vi "oa_Reset if Parameters Change for Triggered Even Angle Signal (N Channels).vi"(7 "reset? (T)":bool=TRUE, 8 "block size":i32=-1, 9 "trigger period [rev]":dbl=1.0, 11 "even angle signals":cluster{"r0":dbl, "dr":dbl, "Y":dbl[]}[](array[cluster]) {"r0" format="%.2p"; "dr" format="%.2p"; "Y" format="%.2f"}) -> (0 "block size out":i32, 1 "trigger period out [rev]":dbl, 3 "even angle signals out":cluster{"r0":dbl, "dr":dbl, "Y":dbl[]}[](array[cluster]) {"r0" format="%.2p"; "dr" format="%.2p"; "Y" format="%.2f"}, 5 "reset out":bool)   [LabVIEW 2017, in "SoundVib_OAUtility.lvlib"]
uses:
  <vilib>/addons/Sound and Vibration/Order Analysis/Utility/SoundVib_OAUtility.lvlib
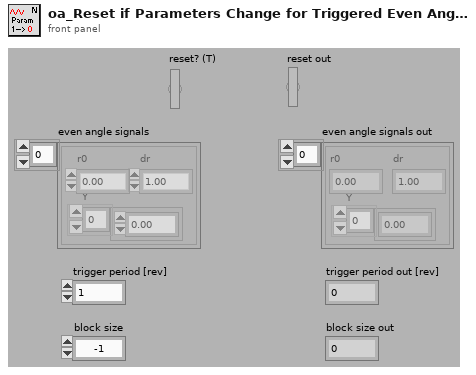
[diagram p1: front panel]
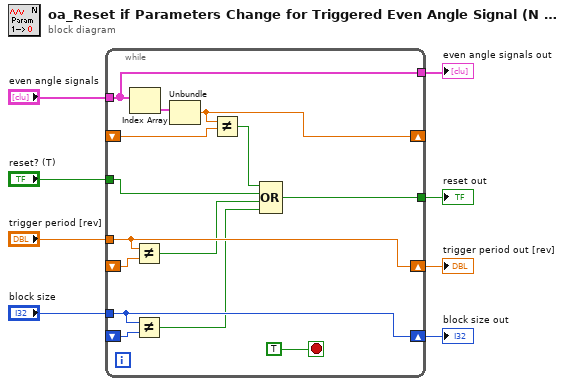
[diagram p0: block diagram]
diagram:
  n1 = while {
    tunnel: "even angle signals" -> [w9]
    shift-right: [w16] -> _
    shift-left: _ -> [w15]
    tunnel: "trigger period [rev]" -> [w20]
    shift-right: [w20] -> w3
    shift-left: _ -> [w19]
    tunnel: "block size" -> [w18]
    shift-right: [w18] -> w2
    shift-left: _ -> [w17]
    tunnel: "reset? (T)" -> [w13]
    tunnel: [w10] -> w4
    tunnel: [w9] -> w1
    stop <- TRUE stop-if-true
    n2 = Index Array(array=w9) -> (element=w21:cluster{"r0":dbl, "dr":dbl, "Y":dbl[]})  [unwired: 1 in]
    n3 = Not Equal?(x=w20, y=w19) -> (x != y?=w12:bool)
    n4 = Not Equal?(x=w18, y=w17) -> (x != y?=w11:bool)
    n5 = Unbundle(w21) -> ("dr"=w16:dbl)  [unwired: 2 out]
    n6 = Not Equal?(x=w16, y=w15) -> (x != y?=w14:bool)
    n7 = Compound Arithmetic op=OR(w14, w13, w12, w11) -> (w10:bool)
  }
  "reset out" <- w4
  "trigger period out [rev]" <- w3
  "block size out" <- w2
  "even angle signals out" <- w1
